vi "EXA shm issue Command EX Ample LV.vi"(8 "error in (no error)":errorcluster, 11 "command_EXAmple_Ctl":cluster{"param1":dbl, "param2":dbl}) -> (0 "error out":errorcluster, 2 "function return":i32, 3 "command_EXAmple_Ctl out":cluster{"param1":dbl, "param2":dbl})   [LabVIEW 2016, in "SALLV_EXA.lvlib"]
doc: "int EXA_shm_issueCommand_EXAmpleLV(EXA_command_EXAmpleLV *command_EXAmple_Ctl );"
uses:
  SALLV_EXA.lvlib
  SALLV_EXA.so
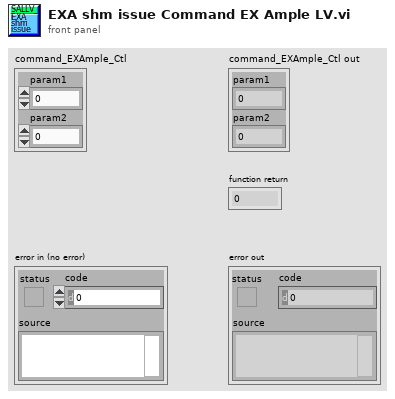
[diagram p1: front panel]
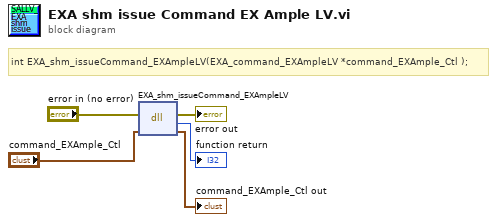
[diagram p0: block diagram]
diagram:
  # "int EXA_shm_issueCommand_EXAmpleLV(EXA_command_EXAmpleLV *command_EXAmple_Ctl );"
  n1 = dll-call lib="home/plotz/SALLV_EXA/SALLV_EXA.*" fn="EXA_shm_issueCommand_EXAmpleLV"(error in="error in (no error)", "command_EXAmple_Ctl"="command_EXAmple_Ctl") -> (error out=→"error out":errorcluster, →"function return":i32, "command_EXAmple_Ctl"=→"command_EXAmple_Ctl out":cluster{"param1":dbl, "param2":dbl})  [unwired: 2 in, 1 out]
